vi "observacao_0MQ.vi"() -> ()   [LabVIEW 2012, in "Shared_160.lvlib"] (continued)
                  }
                }
                n2306 = case shown="True" w2937 {
                  tunnel: w2938 -> [_ w2940]
                  frame False {
                  }
                  frame True {
                    w2943 = u16 4 items=["ZERO", "AH", "DEC", "TUBO", "CUP"] ("Controlador")
                    n2307 = global write "Global_Telescopio.vi" "RevCupTO"(w2940) -> ()
                    n2308 = local write "StatDome"("Waiting" ("Status")) -> ()
                    n2309 = call "Monta Comando.vi"("Comando"="PARAR", "Dispositivo"="PROG", "Controlador"=w2943) -> ()  [unwired: 4 in, 3 out]
                  }
                }
              }
              frame Disabled {
                # "20240820"
                n2310 = global read "Global_Telescopio.vi" "RevCupTO"() -> (w2946:u32)
                n2311 = global read "Global_Telescopio.vi" "QtdEtiquetas"() -> (w2953:i16)
                n2312 = local read "DestCUP"() -> (w2952:i16)
                n2313 = Divide(x=w2953, y=2) -> (x/y=w2951:dbl)
                n2314 = call "TickTimeout.vi"("msInicial"=w2946, "msTimeout"=u32 3000) -> ("msTick"=w2949:u32, "Timeout"=w2948:bool)  [unwired: 1 out]
                n2315 = Subtract(x=w2952, y=w2951) -> (x-y=w2954:dbl)
                n2316 = Add(x=w2952, y=w2951) -> (x+y=w2955:dbl)
                n2317 = Greater?(x=w2955, y=w2953) -> (0:w2956:bool)
                n2318 = Select(t=w2954, s=w2956, f=w2955) -> (s? t:f=w2957:dbl)
                n2319 = case shown="True" w2948 {
                  tunnel: w2949 -> [_ w2964]
                  tunnel: w2957 -> [_ w2959]
                  frame False {
                  }
                  frame True {
                    w2963 = u16 4 items=["ZERO", "AH", "DEC", "TUBO", "CUP"] ("Controlador")
                    n2320 = To Word Integer(number=w2959) -> (16bit integer=w2958:i16)
                    n2321 = global write "Global_Telescopio.vi" "RevCupTO"(w2964) -> ()
                    n2322 = Number To Decimal String(number=w2958) -> (decimal integer string=w2961:string)  [unwired: 1 in]
                    n2323 = local write "StatDome"("Reverting" ("Status")) -> ()
                    n2324 = call "Monta Comando.vi"("Set Point"=w2961, "Comando"="MOVER" ("Dispositivo"), "Dispositivo"="DOMO", "Controlador"=w2963) -> ()  [unwired: 3 in, 3 out]
                  }
                }
              }
              frame Disabled {
                # "20240820"
                n2325 = global read "Global_Telescopio.vi" "RevCupTO"() -> (w2966:u32)
                n2326 = call "TickTimeout.vi"("msInicial"=w2966, "msTimeout"=u32 10000) -> ("msTick"=w2969:u32, "Timeout"=w2968:bool)  [unwired: 1 out]
                n2327 = case shown="True" w2968 {
                  tunnel: w2969 -> [_ w2970]
                  frame False {
                  }
                  frame True {
                    w2973 = u16 4 items=["ZERO", "AH", "DEC", "TUBO", "CUP"] ("Controlador")
                    n2328 = global write "Global_Telescopio.vi" "RevCupTO"(w2970) -> ()
                    n2329 = local write "StatDome"("Wait2s" ("Status")) -> ()
                    n2330 = call "Monta Comando.vi"("Comando"="PARAR", "Dispositivo"="PROG", "Controlador"=w2973) -> ()  [unwired: 4 in, 3 out]
                  }
                }
              }
              frame Disabled {
                n2331 = global read "Global_Telescopio.vi" "RevCupTO"() -> (w2975:u32)
                n2332 = call "TickTimeout.vi"("msInicial"=w2975, "msTimeout"=u32 2000) -> ("msTick"=w2978:u32, "Timeout"=w2977:bool)  [unwired: 1 out]
                n2333 = case shown="True" w2977 {
                  tunnel: w2978 -> [_ w2979]
                  frame False {
                  }
                  frame True {
                    n2334 = global write "Global_Telescopio.vi" "RevCupTO"(w2979) -> ()
                    n2335 = local write "StatDome"("Not Ready" ("Status")) -> ()
                  }
                }
              }
              frame Enabled {
              }
            }
            n2336 = global read "Global_Telescopio.vi" "Telescopio"() -> (w2917:bool)
            n2337 = local read "StatShutter"() -> (w2925:string)
            n2338 = local read "StatDome"() -> (w2927:string)
            n2339 = Select(t=1, s=w2917, f=2) -> (s? t:f=w2915:i32)
            n2340 = event shown="[2] \"BtDomeSTOP\": Value Change" {
              selector: _ -> [_ _ _ _ _ _ _ _]
              dyn-events: _ -> [_ _ _ _ _ _ _ _]
              timeout: 10 -> [_ _ _ _ _ _ _ _]
              tunnel: [FALSE ("NewVal") w3073 w3086 FALSE ("NewVal") FALSE ("NewVal") _ _ _] -> w2924
              tunnel: w2915 -> [_ w3072 _ _ _ _ _ _]
              event Timeout {
                n2341 = event-data() -> ()  [unwired: 1 in, 2 out]
              }
              event "BtDomeGO": Value Change {
                n2342 = event-data() -> ("NewVal"=w3074:bool)  [unwired: 1 in, 5 out]
                n2343 = local read "StatDome"() -> (w3077:string)
                n2344 = Equal?(x=w3077, y="Stopped" ("Status")) -> (x = y?=w3075:bool)
                n2345 = And(x=w3074, y=w3075) -> (x .and. y?=w3073:bool)
                n2346 = case shown="True" w3073 {
                  tunnel: w3072 -> [_ w3081]
                  frame False {
                  }
                  frame True {
                    # "20240820"
                    n2347 = local read "DomeNewPos"() -> (w3078:i32)
                    n2348 = Multiply(x=w3078, y=w3081) -> (x*y=w3079:i32)
                    n2349 = call "Checa destino cupula.vi"("Target"=w3079) -> ("moverCup"=w3080:bool)  [unwired: 6 in, 2 out]
                    n2350 = case shown="True" w3080 {
                      tunnel: w3079 -> [_ w3084]
                      frame False {
                      }
                      frame True {
                        # "Desabilita todas Abas"
                        n2351 = local write "DestCUP"(w3084) -> ()
                        n2352 = local write "DOME"(FALSE) -> ()
                        n2353 = property on="Setup, Pointing & Guiding" class="TabCtl (strict)"("Page Selector Visible"=FALSE) -> ()  [unwired: 2 in, 2 out]
                        n2354 = local write "StatDome"("Not Ready" ("Status")) -> ()
                      }
                    }
                  }
                }
              }
              event "BtDomeSTOP": Value Change {
                n2355 = event-data() -> ("NewVal"=w3086:bool)  [unwired: 1 in, 5 out]
                n2356 = case shown="True" w3086 {
                  frame False {
                  }
                  frame True {
                    n2357 = local read "StatDome"() -> (w3087:string)
                    n2358 = case shown="\"Moving\", Default" w3087 {
                      frame "Stopped" {
                      }
                      frame "Moving", Default {
                        w3088 = u16 4 items=["ZERO", "AH", "DEC", "TUBO", "CUP"] ("Controlador")
                        n2359 = local write "StatDome"("Stopping" ("Status")) -> ()
                        n2360 = call "Monta Comando.vi"("Comando"="PARAR", "Dispositivo"="PROG", "Controlador"=w3088) -> ()  [unwired: 4 in, 3 out]
                      }
                      frame "Not Ready" {
                        n2361 = local write "StatDome"("Stopped" ("Status")) -> ()
                      }
                    }
                  }
                }
              }
              event "BtShutOpen": Value Change {
                n2362 = event-data() -> ("NewVal"=w3095:bool)  [unwired: 1 in, 5 out]
                n2363 = local read "StatShutter"() -> (w3093:string)
                n2364 = case shown="True" w3095 {
                  tunnel: w3093 -> [_ w3096]
                  frame False {
                  }
                  frame True {
                    n2365 = case shown="\"Closed\"" w3096 {
                      frame "Opened", Default {
                      }
                      frame "Closed" {
                        w3097 = FALSE ("WeakSel")
                        w3098 = FALSE ("Coude")
                        w3099 = T5."Enabled" ("Disabled")
                        n2366 = property on="Coude" class="Bool (strict)"("DisabledEnum"=w3099) -> ()  [unwired: 2 in, 2 out]
                        n2367 = property on="Weak" class="Bool (strict)"("Disabled"=w3099) -> ()  [unwired: 2 in, 2 out]
                        n2368 = property on="Medium" class="Bool (strict)"("Disabled"=w3099) -> ()  [unwired: 2 in, 2 out]
                        n2369 = property on="Strong" class="Bool (strict)"("Disabled"=w3099) -> ()  [unwired: 2 in, 2 out]
                        n2370 = local write "StatShutter"("Busy to Open" ("Status")) -> ()
                        n2371 = local write "WeakSel"(w3097) -> ()
                        n2372 = local write "MediumSel"(w3097) -> ()
                        n2373 = local write "Coude"(w3098) -> ()
                        n2374 = local write "Weak"(w3098) -> ()
                        n2375 = local write "Medium"(w3098) -> ()
                        n2376 = local write "Strong"(w3098) -> ()
                        n2377 = local write "StrongSel"(w3097) -> ()
                        n2378 = local write "CoudeSel"(w3097) -> ()
                        n2379 = stacked-sequence {
                          frame #0 {
                            w3102 = u16 4 items=["ZERO", "AH", "DEC", "TUBO", "CUP"] ("Controlador")
                            n2380 = call "Monta Comando.vi"("Comando"="DESLIGAR", "Dispositivo"="FLAT_WEAK", "Controlador"=w3102) -> ()  [unwired: 4 in, 3 out]
                          }
                          frame #1 {
                            w3105 = u16 4 items=["ZERO", "AH", "DEC", "TUBO", "CUP"] ("Controlador")
                            n2381 = call "Monta Comando.vi"("Comando"="DESLIGAR", "Dispositivo"="FLAT_LO", "Controlador"=w3105) -> ()  [unwired: 4 in, 3 out]
                          }
                          frame #2 {
                            w3108 = u16 4 items=["ZERO", "AH", "DEC", "TUBO", "CUP"] ("Controlador")
                            n2382 = call "Monta Comando.vi"("Comando"="DESLIGAR", "Dispositivo"="FLAT_HI", "Controlador"=w3108) -> ()  [unwired: 4 in, 3 out]
                          }
                          frame #3 {
                            w3110 = u16 4 items=["ZERO", "AH", "DEC", "TUBO", "CUP"] ("Controlador")
                            n2383 = call "Monta Comando.vi"("Comando"="DESLIGAR", "Dispositivo"="FLAT_COUDE", "Controlador"=w3110) -> ()  [unwired: 4 in, 3 out]
                          }
                        }
                      }
                    }
                  }
                }
              }
              event "BtShutClose": Value Change {
                n2384 = event-data() -> ("NewVal"=w3114:bool)  [unwired: 1 in, 5 out]
                n2385 = case shown="True" w3114 {
                  frame False {
                  }
                  frame True {
                    n2386 = stacked-sequence {
                      frame #0 {
                        # "MUDANÇA:\nRemovido CASE que não setava essas\nvariáveis se StatShutter = Closed para\ngarantir fechamento da Trapeira."
                        n2387 = local write "DOME"(FALSE) -> ()
                        n2388 = local write "StatShutter"("Busy to Close" ("Status")) -> ()
                      }
                      frame #1 {
                        # "Escreve no LOG o estado do shutter"
                        # "Timer para escrever no log\ne enviar comando:\nCUP TRAPEIRA PARAR"
                        n2389 = Tick Count (ms)() -> (millisecond timer value=w3117:u32)
                        n2390 = local write "shutterTimeOld"(w3117) -> ()
                        n2391 = local write "timeStatShutterAlert"(w3117) -> ()
                        n2392 = local write "sendCommandShutter"(TRUE ("writeShutterLog")) -> ()
                        n2393 = call "Log_Shutter.vi"("command"=" ", "domeState"="CLOSED " ("command"), "pathLogDomeFile"="C:\\TCS\\LOG\\SHUTTER\\SHUTTER.TXT" ("pathLogFocoString")) -> ()  [unwired: 6 in]
                      }
                    }
                  }
                }
              }
              event "BtParavUp": Value Change {
                n2394 = event-data() -> ("NewVal"=w3122:bool)  [unwired: 1 in, 5 out]
                n2395 = case shown="True" w3122 {
                  frame False {
                  }
                  frame True {
                    w3125 = u16 4 items=["ZERO", "AH", "DEC", "TUBO", "CUP"] ("Controlador")
                    n2396 = call "Monta Comando.vi"("Comando"="SUBIR", "Dispositivo"="PARAVENTO" ("Comando"), "Controlador"=w3125) -> ()  [unwired: 4 in, 3 out]
                  }
                }
              }
              event "BtParavDown": Value Change {
                n2397 = event-data() -> ("NewVal"=w3126:bool)  [unwired: 1 in, 5 out]
                n2398 = case shown="True" w3126 {
                  frame False {
                  }
                  frame True {
                    w3129 = u16 4 items=["ZERO", "AH", "DEC", "TUBO", "CUP"] ("Controlador")
                    n2399 = call "Monta Comando.vi"("Comando"="DESCER", "Dispositivo"="PARAVENTO" ("Comando"), "Controlador"=w3129) -> ()  [unwired: 4 in, 3 out]
                  }
                }
              }
              event "BtParavStop": Value Change {
                n2400 = event-data() -> ("NewVal"=w3130:bool)  [unwired: 1 in, 5 out]
                n2401 = case shown="True" w3130 {
                  frame False {
                  }
                  frame True {
                    w3133 = u16 4 items=["ZERO", "AH", "DEC", "TUBO", "CUP"] ("Controlador")
                    n2402 = call "Monta Comando.vi"("Comando"="PARAR", "Dispositivo"="PARAVENTO" ("Comando"), "Controlador"=w3133) -> ()  [unwired: 4 in, 3 out]
                  }
                }
              }
            }
            n2403 = call "Bit Status CUP.vi"("NomeStatus"=w2926) -> ("StatBit"=w2923:bool)
            n2404 = global read "Global_Telescopio.vi" "PosCUP"() -> (w2919:i16)
            n2405 = case shown="\"Moving\"" w2927 {
              tunnel: w2923 -> [_ _ w3062 w3068]
              tunnel: w2924 -> [_ _ _ _]
              frame "", Default {
              }
              frame "Not Ready" {
                n2406 = local read "DestCUP"() -> (w3048:i16)
                n2407 = global read "Global_Telescopio.vi" "PosCUP"() -> (w3050:i16)
                n2408 = call "TickTimeout.vi"() -> ("msTick"=w3051:u32)  [unwired: 2 in, 2 out]
                n2409 = call "Checa destino cupula.vi"("Target"=w3048) -> ("moverCup"=w3047:bool, "angTarget"=w3049:string)  [unwired: 6 in, 1 out]
                n2410 = case shown="True" w3047 {
                  tunnel: w3051 -> [_ w3057]
                  tunnel: w3050 -> [_ w3056]
                  tunnel: w3049 -> [_ w3055]
                  tunnel: w3048 -> [_ w3054]
                  frame False {
                    n2411 = local write "StatDome"("Stopping" ("Status")) -> ()
                  }
                  frame True {
                    w3061 = u16 4 items=["ZERO", "AH", "DEC", "TUBO", "CUP"] ("Controlador")
                    # "20240820"
                    n2412 = global write "Global_Telescopio.vi" "RevCupTO"(w3057) -> ()
                    n2413 = local write "TargetCup"(w3055) -> ()
                    n2414 = global write "Global_Telescopio.vi" "CupStartPos"(w3056) -> ()
                    n2415 = Number To Decimal String(number=w3054) -> (decimal integer string=w3058:string)  [unwired: 1 in]
                    n2416 = local write "StatDome"("Moving" ("Status")) -> ()
                    n2417 = call "Monta Comando.vi"("Set Point"=w3058, "Comando"="MOVER", "Dispositivo"="DOMO" ("Comando"), "Controlador"=w3061) -> ()  [unwired: 3 in, 3 out]
                  }
                }
              }
              frame "Moving" {
                n2418 = case shown="False" w3062 {
                  frame False {
                    n2419 = local read "DestCUP"() -> (w3067:i16)
                    n2420 = call "Checa destino cupula.vi"("Target"=w3067) -> ("moverCup"=w3066:bool)  [unwired: 6 in, 2 out]
                    n2421 = Select(t="Not Ready" ("Comando"), s=w3066, f="Stopping" ("Comando")) -> (s? t:f=w3065:string)
                    n2422 = local write "StatDome"(w3065) -> ()
                  }
                  frame True {
                  }
                }
              }
              frame "Stopping" {
                n2423 = case shown="False" w3068 {
                  frame False {
                    # "Reabilita Abas"
                    n2424 = property on="Setup, Pointing & Guiding" class="TabCtl (strict)"("Page Selector Visible"=TRUE) -> ()  [unwired: 2 in, 2 out]
                    n2425 = local write "StatDome"("Stopped" ("Status")) -> ()
                  }
                  frame True {
                  }
                }
              }
            }
            n2426 = call "Bit Status CUP.vi"("NomeStatus"=w2922) -> ("StatBit"=w2921:bool)
            "LedShutter" <- w2921
            n2427 = case shown="\"Busy to Close\"" w2925 {
              tunnel: w2924 -> [_ _ _ _]
              tunnel: w2923 -> [_ w3030 w3036 _]
              frame "", Default {
              }
              frame "Busy to Open" {
                n2428 = case shown="False" w3030 {
                  frame False {
                    w3034 = u16 4 items=["ZERO", "AH", "DEC", "TUBO", "CUP"] ("Controlador")
                    n2429 = call "TickTimeout.vi"() -> ("msTick"=w3031:u32)  [unwired: 2 in, 2 out]
                    n2430 = local write "TimeoutTrap"(w3031) -> ()
                    n2431 = local write "StatShutter"("Moving" ("Status")) -> ()
                    n2432 = call "Monta Comando.vi"("Comando"="ABRIR", "Dispositivo"="TRAPEIRA" ("Comando"), "Controlador"=w3034) -> ()  [unwired: 4 in, 3 out]
                  }
                  frame True {
                  }
                }
              }
              frame "Busy to Close" {
                n2433 = case shown="False" w3036 {
                  frame False {
                    w3040 = u16 4 items=["ZERO", "AH", "DEC", "TUBO", "CUP"] ("Controlador")
                    n2434 = call "TickTimeout.vi"() -> ("msTick"=w3037:u32)  [unwired: 2 in, 2 out]
                    n2435 = local write "TimeoutTrap"(w3037) -> ()
                    n2436 = local write "StatShutter"("Moving" ("Status")) -> ()
                    n2437 = call "Monta Comando.vi"("Comando"="FECHAR", "Dispositivo"="TRAPEIRA" ("Comando"), "Controlador"=w3040) -> ()  [unwired: 4 in, 3 out]
                  }
                  frame True {
                  }
                }
              }
              frame "Moving" {
                n2438 = local read "TimeoutTrap"() -> (w3042:u32)
                n2439 = call "TickTimeout.vi"("msInicial"=w3042, "msTimeout"=u32 12000) -> ("Timeout"=w3043:bool)  [unwired: 2 out]
                n2440 = case shown="False" w3043 {
                  selector: w3043 -> [w3046 _]
                  frame False {
                    n2441 = Not(x=w3046) -> (.not. x?=w3045:bool)
                    n2442 = local write "RefreshShutterState"(w3045) -> ()
                  }
                  frame True {
                  }
                }
              }
            }
            n2443 = local read "RefreshShutterState"() -> (w2920:bool)
            n2444 = Divide(x=w2919, y=w2915) -> (x/y=w2930:dbl)
            n2445 = To Word Integer(number=w2930) -> (16bit integer=→"AngCup":i16)
            n2446 = case shown="True" w2920 {
              selector: w2920 -> [_ w3025]
              tunnel: w2921 -> [_ w3026]
              frame False {
              }
              frame True {
                n2447 = Not(x=w3025) -> (.not. x?=→"RefreshShutterState":bool)
                n2448 = Select(t="Opened" ("Status"), s=w3026, f="Closed" ("Status")) -> (s? t:f=w3027:string)
                n2449 = local write "StatShutter"(w3027) -> ()
              }
            }
            n2450 = local read "Flag-ShutClose"() -> (w2913:bool)
            n2451 = local read "Flag-ShutOpen"() -> (w2912:bool)
            n2452 = event shown="[1] \"BtShutClose\": Value Change" {
              selector: _ -> [_ _ _]
              dyn-events: _ -> [_ _ _]
              timeout: 10 -> [_ _ _]
              event Timeout {
                n2453 = event-data() -> ()  [unwired: 1 in, 2 out]
              }
              event "BtShutClose": Value Change {
                # "Desabilita todas Abas"
                n2454 = event-data() -> ("NewVal"=w3006:bool)  [unwired: 1 in, 4 out]
                n2455 = case shown="True" w3006 {
                  selector: w3006 -> [_ w3011]
                  frame False {
                  }
                  frame True {
                    n2456 = Get Date/Time In Seconds() -> (seconds since 1Jan1904=w3010:timestamp)
                    n2457 = Add(x=w3010, y=10.0) -> (x+y=w3008:timestamp)
                    n2458 = local write "Cont-ShutOpen"(w3008) -> ()
                    n2459 = property on="Setup, Pointing & Guiding" class="TabCtl (strict)"("Page Selector Visible"=FALSE) -> ()  [unwired: 2 in, 2 out]
                    "Flag-ShutClose" <- w3011
                  }
                }
              }
              event "BtShutOpen": Value Change {
                # "Desabilita todas Abas"
                n2460 = event-data() -> ("NewVal"=w3012:bool)  [unwired: 1 in, 4 out]
                n2461 = case shown="True" w3012 {
                  selector: w3012 -> [_ w3013]
                  frame False {
                  }
                  frame True {
                    n2462 = stacked-sequence {
                      tunnel: w3013 -> [w3018 _]
                      frame #0 {
                        n2463 = Get Date/Time In Seconds() -> (seconds since 1Jan1904=w3017:timestamp)
                        n2464 = Add(x=w3017, y=10.0) -> (x+y=→"Cont-ShutOpen":timestamp)
                        n2465 = property on="Setup, Pointing & Guiding" class="TabCtl (strict)"("Page Selector Visible"=FALSE) -> ()  [unwired: 2 in, 2 out]
                        "Flag-ShutOpen" <- w3018
                      }
                      frame #1 {
                        # "Escreve no LOG o estado do shutter"
                        # "Timer para escrever no log\ne enviar comando:\nCUP TRAPEIRA PARAR"
                        n2466 = Tick Count (ms)() -> (millisecond timer value=w3019:u32)
                        n2467 = local write "sendCommandShutter"(TRUE ("writeShutterLog")) -> ()
                        n2468 = local write "timeStatShutterAlert"(w3019) -> ()
                        n2469 = local write "shutterTimeOld"(w3019) -> ()
                        n2470 = call "Log_Shutter.vi"("command"=" ", "domeState"="OPENED " ("command"), "pathLogDomeFile"="C:\\TCS\\LOG\\SHUTTER\\SHUTTER.TXT" ("pathLogFocoString")) -> ()  [unwired: 6 in]
                      }
                    }
                  }
                }
              }
            }
            n2471 = event shown="[4] \"CW\": Mouse Up" {
              selector: _ -> [_ _ _ _ _]
              dyn-events: _ -> [_ _ _ _ _]
              timeout: 100 -> [_ _ _ _ _]
              event Timeout {
                n2472 = event-data() -> ()  [unwired: 1 in, 2 out]
              }
              event "CCW": Mouse Down {
                w2981 = "GIRAR_CCW" ("Comando")
                w2982 = u16 4 items=["ZERO", "AH", "DEC", "TUBO", "CUP"] ("Controlador")
                # "Envia o comando GIRAR"
                n2473 = event-data() -> ()  [unwired: 1 in, 7 out]
                n2474 = local write "Command"(w2981) -> ()
                n2475 = call "Monta Comando.vi"("Comando"=w2981, "Dispositivo"="DOMO" ("Comando"), "Controlador"=w2982) -> ()  [unwired: 4 in, 3 out]
              }
              event "CCW": Mouse Up {
                n2476 = event-data() -> ()  [unwired: 1 in, 7 out]
                n2477 = stacked-sequence {
                  frame #0 {
                    w2984 = "PARAR" ("Comando")
                    w2985 = u16 4 items=["ZERO", "AH", "DEC", "TUBO", "CUP"] ("Controlador")
                    # "Envia o comando PARAR"
                    n2478 = local write "Command"(w2984) -> ()
                    n2479 = call "Monta Comando.vi"("Comando"=w2984, "Dispositivo"="DOMO" ("Comando"), "Controlador"=w2985) -> ()  [unwired: 4 in, 3 out]
                  }
                  frame #1 {
                    n2480 = Wait (ms)(milliseconds to wait=u32 100) -> ()  [unwired: 1 out]
                  }
                  frame #2 {
                    w2988 = "PARAR" ("Comando")
                    w2989 = u16 4 items=["ZERO", "AH", "DEC", "TUBO", "CUP"] ("Controlador")
                    # "Envia o comando PARAR"
                    n2481 = local write "Command"(w2988) -> ()
                    n2482 = call "Monta Comando.vi"("Comando"=w2988, "Dispositivo"="DOMO" ("Comando"), "Controlador"=w2989) -> ()  [unwired: 4 in, 3 out]
                  }
                }
              }
              event "CW": Mouse Down {
                w2991 = "GIRAR_CW" ("Comando")
                w2992 = u16 4 items=["ZERO", "AH", "DEC", "TUBO", "CUP"] ("Controlador")
                # "Envia o comando GIRAR"
                n2483 = event-data() -> ()  [unwired: 1 in, 7 out]
                n2484 = local write "Command"(w2991) -> ()
                n2485 = call "Monta Comando.vi"("Comando"=w2991, "Dispositivo"="DOMO" ("Comando"), "Controlador"=w2992) -> ()  [unwired: 4 in, 3 out]
              }
              event "CW": Mouse Up {
                n2486 = event-data() -> ()  [unwired: 1 in, 7 out]
                n2487 = stacked-sequence {
                  frame #0 {
                    w2994 = "PARAR" ("Comando")
                    w2995 = u16 4 items=["ZERO", "AH", "DEC", "TUBO", "CUP"] ("Controlador")
                    # "Envia o comando PARAR"
                    n2488 = local write "Command"(w2994) -> ()
                    n2489 = call "Monta Comando.vi"("Comando"=w2994, "Dispositivo"="DOMO" ("Comando"), "Controlador"=w2995) -> ()  [unwired: 4 in, 3 out]
                  }
                  frame #1 {
                    n2490 = Wait (ms)(milliseconds to wait=u32 100) -> ()  [unwired: 1 out]
                  }
                  frame #2 {
                    w2998 = "PARAR" ("Comando")
                    w2999 = u16 4 items=["ZERO", "AH", "DEC", "TUBO", "CUP"] ("Controlador")
                    # "Envia o comando PARAR"
                    n2491 = local write "Command"(w2998) -> ()
                    n2492 = call "Monta Comando.vi"("Comando"=w2998, "Dispositivo"="DOMO" ("Comando"), "Controlador"=w2999) -> ()  [unwired: 4 in, 3 out]
                  }
                }
              }
            }
            n2493 = Or(x=w2913, y=w2912) -> (x .or. y?=w2911:bool)
            n2494 = case shown="True" w2911 {
              frame False {
              }
              frame True {
                n2495 = local read "Cont-ShutOpen"() -> (w3002:timestamp)
                n2496 = Get Date/Time In Seconds() -> (seconds since 1Jan1904=w3003:timestamp)
                n2497 = Greater Or Equal?(x=w3003, y=w3002) -> (x >= y?=w3001:bool)
                n2498 = case shown="True" w3001 {
                  frame False {
                  }
                  frame True {
                    w3005 = FALSE ("Flag-ShutClose")
                    # "Reabilita todas Abas"
                    n2499 = local write "Flag-ShutClose"(w3005) -> ()
                    n2500 = local write "Flag-ShutOpen"(w3005) -> ()
                    n2501 = property on="Setup, Pointing & Guiding" class="TabCtl (strict)"("Page Selector Visible"=TRUE) -> ()  [unwired: 2 in, 2 out]
                  }
                }
              }
            }
            "Command" <- "" ("Command")
          }
          frame "UTILS " {
            n2502 = stacked-sequence {
              frame #0 {
                # "Acionamento das Abas do\nEspelho\n\nComandos sempre precedidos\nde ESPAÇO\n\nTUBO TAMPAS ESCREVER = 80 80\n\nLigar power geral       08 08\nDesligar power geral  08 00\nLigar System              10 10\nDesligar System         10 00\nPassar para Remoto  20 20\nPassar para Local      20 00\nSel. device central     40 40\nSel. device bowl         40 00\nAction open                80 80\nAction close                80 00"
                n2503 = event shown="[1] \"MODE\": Value Change" {
                  selector: _ -> [_ _ _]
                  dyn-events: _ -> [_ _ _]
                  timeout: 10 -> [_ _ _]
                  event Timeout {
                    n2504 = event-data() -> ()  [unwired: 1 in, 2 out]
                  }
                  event "MODE": Value Change {
                    n2505 = event-data() -> ("NewVal"=w3148:bool)  [unwired: 1 in, 5 out]
                    "LED MODE" <- w3148
                    n2506 = case shown="False" w3148 {
                      frame False {
                        w3153 = u16 3 items=["ZERO", "AH", "DEC", "TUBO", "CUP"] ("Controlador")
                        # "DESABILITA"
                        # "APENAS PASSANDO COMANDO PARA MANETE"
                        # "MODE E GERAL = 0"
                        # "MODE HADSET"
                        n2507 = call "Monta Comando.vi"("Set Point"=" F8 90", "Comando"="ESCREVER", "Dispositivo"="TAMPAS" ("Comando"), "Controlador"=w3153) -> ()  [unwired: 3 in, 3 out]
                        n2508 = property on="ACTION" class="Bool (strict)"("Disabled"=u8 2) -> ()  [unwired: 2 in, 2 out]
                      }
                      frame True {
                        w3158 = u16 3 items=["ZERO", "AH", "DEC", "TUBO", "CUP"] ("Controlador")
                        # "HABILITA"
                        # "APENAS PASSANDO COMOANDO PARA TCSPD"
                        # "MODE E GERAL = 1"
                        # "MODE TCSPD"
                        n2509 = call "Monta Comando.vi"("Set Point"=" 48 48", "Comando"="ESCREVER", "Dispositivo"="TAMPAS" ("Comando"), "Controlador"=w3158) -> ()  [unwired: 3 in, 3 out]
                        n2510 = property on="ACTION" class="Bool (strict)"("Disabled"=u8 0) -> ()  [unwired: 2 in, 2 out]
                      }
                    }
                  }
                  event "ACTION": Value Change {
                    n2511 = event-data() -> ("NewVal"=w3159:bool)  [unwired: 1 in, 5 out]
                    n2512 = case shown="False" w3159 {
                      frame False {
                        # "FECHAR"
                        n2513 = local write "ESTADO FECHAR"("INICIO" ("ESTADO ABRIR")) -> ()
                        n2514 = local write "ESTADO ABRIR"("REPOUSO" ("ESTADO ABRIR")) -> ()
                      }
                      frame True {
                        # "ABRIR"
                        n2515 = local write "ESTADO FECHAR"("REPOUSO" ("ESTADO ABRIR")) -> ()
                        n2516 = local write "ESTADO ABRIR"("INICIO" ("ESTADO ABRIR")) -> ()
                      }
                    }
                  }
                }
                n2517 = Tick Count (ms)() -> (millisecond timer value=w3139:u32)
                n2518 = Greater Or Equal?(x=w3139, y="TIMER TICK") -> (x >= y?=w3135:bool)
                n2519 = And(x=w3135, y=FALSE) -> (x .and. y?=w3136:bool)
                n2520 = case shown="True" w3136 {
                  frame False {
                  }
                  frame True {
                    w3172 = u16 3 items=["ZERO", "AH", "DEC", "TUBO", "CUP", "CASS", "COUDE"] ("Controlador")
                    # "2 SEGUNDOS"
                    n2521 = Tick Count (ms)() -> (millisecond timer value=w3169:u32)
                    n2522 = Add(x=w3169, y=u32 10000) -> (x+y=w3167:u32)
                    n2523 = call "Status_das_Tampas.vi"("Controlador"=w3172, "DISPOSITIVO"="TAMPAS", "Comando"="LER") -> ("Fechado/Aberto"=w3166:bool, "Dispositivo Bacia/Centar"=w3165:bool)  [unwired: 6 in, 5 out]
                    n2524 = local write "TIMER TICK"(w3167) -> ()
                    n2525 = Not(x=w3166) -> (.not. x?=w3164:bool)
                    n2526 = And(x=w3164, y=w3165) -> ()  [unwired: 1 out]
                  }
                }
                n2527 = event shown="[4] \"FLAT-FIELD\": Value Change" {
                  selector: _ -> [_ _ _ _ _ _]
                  dyn-events: _ -> [_ _ _ _ _ _]
                  timeout: 10 -> [_ _ _ _ _ _]
                  event Timeout {
                    n2528 = event-data() -> ()  [unwired: 1 in, 2 out]
                  }
                  event "BtUtilPark": Value Change {
                    n2529 = event-data() -> ("NewVal"=w3173:bool)  [unwired: 1 in, 5 out]
                    n2530 = case shown="True" w3173 {
                      frame False {
                      }
                      frame True {
                        w3176 = u16 4 items=["ZERO", "AH", "DEC", "TUBO", "CUP"] ("Controlador")
                        w3177 = FALSE ("MOUNT")
                        w3180 = 0 ("M_AH")
                        w3181 = u8 2 ("Disabled")
                        w3178 = FALSE ("Page Selector Visible")
                        w3185 = 1 ("M_AH")
                        # "Carrega Parâmetros da Configuração"
                        # "Seta Máq GO"
                        # "Desabilita todas Abas"
                        # "DESABILITA TODOS"
                        n2531 = local write "DOME"(w3178) -> ()
                        n2532 = property on="Setup, Pointing & Guiding" class="TabCtl (strict)"("Page Selector Visible"=w3178) -> ()  [unwired: 2 in, 2 out]
                        n2533 = local write "statAH"(w3180) -> ()
                        n2534 = local write "statCUP"(w3180) -> ()
                        n2535 = local write "statDEC"(w3180) -> ()
                        n2536 = local write "M_DEC"(w3185) -> ()
                        n2537 = local write "M_AH"(w3185) -> ()
                        n2538 = local write "M_CUP"(w3185) -> ()
                        n2539 = global read "Global_Telescopio.vi" "DestDEC"() -> (w3183:dbl)
                        n2540 = global read "Global_Telescopio.vi" "DestCUP"() -> (w3182:i32)
                        n2541 = global read "Global_Telescopio.vi" "DestAH"() -> (w3184:dbl)
                        n2542 = property on="BtUtilPark" class="Bool (strict)"("Disabled"=w3181) -> ()  [unwired: 2 in, 2 out]
                        n2543 = property on="ECASS" class="Bool (strict)"("Disabled"=w3181) -> ()  [unwired: 2 in, 2 out]
                        n2544 = local write "DestAH"(w3184) -> ()
                        n2545 = local write "DestCUP"(w3182) -> ()
                        n2546 = local write "DestDEC"(w3183) -> ()
                        n2547 = global write "Global_Telescopio.vi" "Parking"(TRUE ("Page Selector Visible")) -> ()
                        n2548 = property on="BtUtilZenith" class="Bool (strict)"("Disabled"=w3181) -> ()  [unwired: 2 in, 2 out]
                        n2549 = property on="FLAT-FIELD" class="Bool (strict)"("Disabled"=w3181) -> ()  [unwired: 2 in, 2 out]
                        n2550 = property on="PROTEÇÃO" class="Bool (strict)"("Disabled"=w3181) -> ()  [unwired: 2 in, 2 out]
                        n2551 = local write "MOUNT"(w3177) -> ()
                        n2552 = local write "GUIDER"(w3177) -> ()
                        n2553 = call "Monta Comando.vi"("Comando"="LIGAR", "Dispositivo"="LAMP_CAM" ("Comando"), "Controlador"=w3176) -> ()  [unwired: 4 in, 3 out]
                      }
                    }
                  }
                  event "BtUtilZenith": Value Change {
                    n2554 = event-data() -> ("NewVal"=w3186:bool)  [unwired: 1 in, 5 out]
                    n2555 = case shown="True" w3186 {
                      frame False {
                      }
                      frame True {
                        w3189 = u16 4 items=["ZERO", "AH", "DEC", "TUBO", "CUP"] ("Controlador")
                        w3190 = FALSE ("MOUNT")
                        w3193 = 0 ("M_AH")
                        w3194 = u8 2 ("Disabled")
                        w3192 = FALSE ("Page Selector Visible")
                        w3198 = 1 ("M_AH")
                        # "Seta Máq GO"
                        # "Desabilita todas Abas"
                        # "DESABILITA TODOS"
                        n2556 = local write "M_DEC"(w3198) -> ()
                        n2557 = local write "M_AH"(w3198) -> ()
                        n2558 = local write "M_CUP"(w3198) -> ()
                        n2559 = local write "DOME"(w3192) -> ()
                        n2560 = property on="Setup, Pointing & Guiding" class="TabCtl (strict)"("Page Selector Visible"=w3192) -> ()  [unwired: 2 in, 2 out]
                        n2561 = call "Monta Comando.vi"("Comando"="LIGAR", "Dispositivo"="LAMP_CAM" ("Comando"), "Controlador"=w3189) -> ()  [unwired: 4 in, 3 out]
                        n2562 = local write "statAH"(w3193) -> ()
                        n2563 = local write "statCUP"(w3193) -> ()
                        n2564 = local write "statDEC"(w3193) -> ()
                        n2565 = global read "Global_Telescopio.vi" "Telescopio"() -> (w3191:bool)
                        n2566 = property on="BtUtilPark" class="Bool (strict)"("Disabled"=w3194) -> ()  [unwired: 2 in, 2 out]
                        n2567 = property on="ECASS" class="Bool (strict)"("Disabled"=w3194) -> ()  [unwired: 2 in, 2 out]
                        n2568 = case shown="False" w3191 {
                          tunnel: [0.0 ("DestAH") 0.0 ("DestAH")] -> w3197
                          tunnel: [-0.3933 ("DestDEC") -0.3933 ("DestDEC")] -> w3196
                          tunnel: [i16 98 ("DestCUP") i16 80 ("DestCUP")] -> w3195
                          frame False {
                          }
                          frame True {
                          }
                        }
                        n2569 = property on="BtUtilZenith" class="Bool (strict)"("Disabled"=w3194) -> ()  [unwired: 2 in, 2 out]
                        n2570 = property on="FLAT-FIELD" class="Bool (strict)"("Disabled"=w3194) -> ()  [unwired: 2 in, 2 out]
                        n2571 = local write "DestAH"(w3197) -> ()
                        n2572 = local write "DestCUP"(w3195) -> ()
                        n2573 = local write "DestDEC"(w3196) -> ()
                        n2574 = property on="PROTEÇÃO" class="Bool (strict)"("Disabled"=w3194) -> ()  [unwired: 2 in, 2 out]
                        n2575 = local write "MOUNT"(w3190) -> ()
                        n2576 = local write "GUIDER"(w3190) -> ()
                      }
                    }
                  }
                  event "ECASS": Value Change {
                    n2577 = event-data() -> ("NewVal"=w3205:bool)  [unwired: 1 in, 5 out]
                    n2578 = case shown="True" w3205 {
                      frame False {
                      }
                      frame True {
                        w3208 = u16 4 items=["ZERO", "AH", "DEC", "TUBO", "CUP"] ("Controlador")
                        w3209 = FALSE ("MOUNT")
                        w3212 = 0 ("M_AH")
                        w3213 = u8 2 ("Disabled")
                        w3211 = FALSE ("Page Selector Visible")
                        w3217 = 1 ("M_AH")
                        # "Seta Máq GO"
                        # "Desabilita todas Abas"
                        # "DESABILITA TODOS"
                        n2579 = local write "M_DEC"(w3217) -> ()
                        n2580 = local write "M_AH"(w3217) -> ()
                        n2581 = local write "M_CUP"(w3217) -> ()
                        n2582 = local write "DOME"(w3211) -> ()
                        n2583 = property on="Setup, Pointing & Guiding" class="TabCtl (strict)"("Page Selector Visible"=w3211) -> ()  [unwired: 2 in, 2 out]
                        n2584 = local write "statAH"(w3212) -> ()
                        n2585 = local write "statCUP"(w3212) -> ()
                        n2586 = local write "statDEC"(w3212) -> ()
                        n2587 = call "Monta Comando.vi"("Comando"="LIGAR", "Dispositivo"="LAMP_CAM" ("Comando"), "Controlador"=w3208) -> ()  [unwired: 4 in, 3 out]
                        n2588 = global read "Global_Telescopio.vi" "Telescopio"() -> (w3210:bool)
                        n2589 = property on="BtUtilPark" class="Bool (strict)"("Disabled"=w3213) -> ()  [unwired: 2 in, 2 out]
                        n2590 = property on="ECASS" class="Bool (strict)"("Disabled"=w3213) -> ()  [unwired: 2 in, 2 out]
                        n2591 = property on="BtUtilZenith" class="Bool (strict)"("Disabled"=w3213) -> ()  [unwired: 2 in, 2 out]
                        n2592 = property on="FLAT-FIELD" class="Bool (strict)"("Disabled"=w3213) -> ()  [unwired: 2 in, 2 out]
                        n2593 = case shown="False" w3210 {
                          tunnel: [0.0 ("DestAH") 0.0 ("DestAH")] -> w3216
                          tunnel: [0.4 ("DestDEC") 0.4 ("DestDEC")] -> w3215
                          tunnel: [i16 98 ("DestCUP") i16 80 ("DestCUP")] -> w3214
                          frame False {
                          }
                          frame True {
                          }
                        }
                        n2594 = property on="PROTEÇÃO" class="Bool (strict)"("Disabled"=w3213) -> ()  [unwired: 2 in, 2 out]
                        n2595 = local write "GUIDER"(w3209) -> ()
                        n2596 = local write "MOUNT"(w3209) -> ()
                        n2597 = local write "DestAH"(w3216) -> ()
                        n2598 = local write "DestCUP"(w3214) -> ()
                        n2599 = local write "DestDEC"(w3215) -> ()
                      }
                    }
                  }
                  event "FLAT-FIELD": Value Change {
                    n2600 = event-data() -> ("NewVal"=w3224:bool)  [unwired: 1 in, 5 out]
                    n2601 = case shown="True" w3224 {
                      frame False {
                      }
                      frame True {
                        w3227 = u16 4 items=["ZERO", "AH", "DEC", "TUBO", "CUP"] ("Controlador")
                        w3228 = FALSE ("MOUNT")
                        w3230 = 0 ("M_AH")
                        w3232 = u8 2 ("Disabled")
                        w3231 = FALSE ("Page Selector Visible")
                        w3236 = 1 ("M_AH")
                        # "Seta Máq GO"
                        # "Desabilita todas Abas"
                        # "DESABILITA TODOS"
                        n2602 = local write "M_DEC"(w3236) -> ()
                        n2603 = local write "M_AH"(w3236) -> ()
                        n2604 = local write "M_CUP"(w3236) -> ()
                        n2605 = local write "DOME"(w3231) -> ()
                        n2606 = property on="Setup, Pointing & Guiding" class="TabCtl (strict)"("Page Selector Visible"=w3231) -> ()  [unwired: 2 in, 2 out]
                        n2607 = call "Monta Comando.vi"("Comando"="LIGAR", "Dispositivo"="LAMP_CAM" ("Comando"), "Controlador"=w3227) -> ()  [unwired: 4 in, 3 out]
                        n2608 = local write "statAH"(w3230) -> ()
                        n2609 = local write "statCUP"(w3230) -> ()
                        n2610 = local write "statDEC"(w3230) -> ()
                        n2611 = global read "Global_Telescopio.vi" "Telescopio"() -> (w3229:bool)
                        n2612 = property on="BtUtilPark" class="Bool (strict)"("Disabled"=w3232) -> ()  [unwired: 2 in, 2 out]
                        n2613 = property on="ECASS" class="Bool (strict)"("Disabled"=w3232) -> ()  [unwired: 2 in, 2 out]
                        n2614 = case shown="False" w3229 {
                          tunnel: [0.0715 ("DestAH") 0.31416 ("DestAH")] -> w3235
                          tunnel: [0.641 ("DestDEC") -0.39415 ("DestDEC")] -> w3234
                          tunnel: [i16 306 ("DestCUP") i16 133 ("DestCUP")] -> w3233
                          frame False {
                          }
                          frame True {
                          }
                        }
                        n2615 = property on="BtUtilZenith" class="Bool (strict)"("Disabled"=w3232) -> ()  [unwired: 2 in, 2 out]
                        n2616 = property on="FLAT-FIELD" class="Bool (strict)"("Disabled"=w3232) -> ()  [unwired: 2 in, 2 out]
                        n2617 = local write "DestAH"(w3235) -> ()
                        n2618 = local write "DestCUP"(w3233) -> ()
                        n2619 = local write "DestDEC"(w3234) -> ()
                        n2620 = property on="PROTEÇÃO" class="Bool (strict)"("Disabled"=w3232) -> ()  [unwired: 2 in, 2 out]
                        n2621 = local write "GUIDER"(w3228) -> ()
                        n2622 = local write "MOUNT"(w3228) -> ()
                      }
                    }
                  }
                  event "PROTEÇÃO": Value Change {
                    n2623 = event-data() -> ("NewVal"=w3243:bool)  [unwired: 1 in, 5 out]
                    n2624 = case shown="True" w3243 {
                      frame False {
                      }
                      frame True {
                        w3244 = FALSE ("MOUNT")
                        w3246 = 0 ("M_AH")
                        w3245 = FALSE ("Page Selector Visible")
                        w3248 = u8 2 ("Disabled")
                        # "Seta Máq GO"
                        # "Desabilita todas Abas"
                        # "DESABILITA TODOS"
                        n2625 = local write "DOME"(w3245) -> ()
                        n2626 = property on="Setup, Pointing & Guiding" class="TabCtl (strict)"("Page Selector Visible"=w3245) -> ()  [unwired: 2 in, 2 out]
                        n2627 = local write "statAH"(w3246) -> ()
                        n2628 = local write "statCUP"(w3246) -> ()
                        n2629 = local write "statDEC"(w3246) -> ()
                        n2630 = property on="BtUtilPark" class="Bool (strict)"("Disabled"=w3248) -> ()  [unwired: 2 in, 2 out]
                        n2631 = property on="ECASS" class="Bool (strict)"("Disabled"=w3248) -> ()  [unwired: 2 in, 2 out]
                        n2632 = property on="BtUtilZenith" class="Bool (strict)"("Disabled"=w3248) -> ()  [unwired: 2 in, 2 out]
                        n2633 = property on="FLAT-FIELD" class="Bool (strict)"("Disabled"=w3248) -> ()  [unwired: 2 in, 2 out]
                        n2634 = local write "M_PROT"(1 ("M_PROT")) -> ()
                        n2635 = local write "GUIDER"(w3244) -> ()
                        n2636 = local write "MOUNT"(w3244) -> ()
                        n2637 = property on="PROTEÇÃO" class="Bool (strict)"("Disabled"=w3248) -> ()  [unwired: 2 in, 2 out]
                      }
                    }
                  }
                }
                n2638 = case shown="True" "STOP" {
                  frame False {
                  }
                  frame True {
                    n2639 = stacked-sequence {
                      frame #0 {
                        w3250 = 0 ("estado")
                        # "Zera Máquina de Estado\nPelo Botão STOP"
                        n2640 = property on="Setup, Pointing & Guiding" class="TabCtl (strict)"("Page Selector Visible"=TRUE) -> ()  [unwired: 2 in, 2 out]
                        n2641 = call "Stop.vi"() -> ()  [unwired: 1 in, 1 out]
                        n2642 = local write "Flag Stop"(TRUE ("Flag Stop")) -> ()
                        n2643 = local write "M_AH"(w3250) -> ()
                        n2644 = local write "M_DEC"(w3250) -> ()
                        n2645 = local write "M_CUP"(w3250) -> ()
                        n2646 = local write "M_PROT"(w3250) -> ()
                      }
                      frame #1 {
                        w3252 = FALSE
                        w3253 = u8 0 ("Disabled")
                        # "DESLIGA TODOS"
                        # "HABILITA TODOS"
                        n2647 = local write "BtUtilZenith"(w3252) -> ()
                        n2648 = local write "BtUtilPark"(w3252) -> ()
                        n2649 = local write "FLAT-FIELD"(w3252) -> ()
                        n2650 = local write "PROTEÇÃO"(w3252) -> ()
                        n2651 = local write "ECASS"(w3252) -> ()
                        n2652 = property on="BtUtilPark" class="Bool (strict)"("Disabled"=w3253) -> ()  [unwired: 2 in, 2 out]
                        n2653 = property on="ECASS" class="Bool (strict)"("Disabled"=w3253) -> ()  [unwired: 2 in, 2 out]
                        n2654 = property on="BtUtilZenith" class="Bool (strict)"("Disabled"=w3253) -> ()  [unwired: 2 in, 2 out]
                        n2655 = property on="PROTEÇÃO" class="Bool (strict)"("Disabled"=w3253) -> ()  [unwired: 2 in, 2 out]
                        n2656 = property on="FLAT-FIELD" class="Bool (strict)"("Disabled"=w3253) -> ()  [unwired: 2 in, 2 out]
                      }
                    }
                  }
                }
                n2657 = Compound Arithmetic op=OR("BtUtilPark", "BtUtilZenith", "ECASS", "FLAT-FIELD", "PROTEÇÃO") -> (→"MOVING":bool)
              }
              frame #1 {
                # "MÁQUINAS DE ESTADOS DAS TAMPAS"
                n2658 = case shown="True" "Case Constant\n(See Context Help) 11" {
                  frame False {
                    # "ABRIR"
                    # "FECHAR"
                    n2659 = case shown="\"PIZZA\"" "ESTADO FECHAR" {
                      tunnel: [w3304 w3312 w3323 w3331 w3341 w3349 w3359 "REPOUSO" ("y")] -> w3258
                      frame "INICIO", Default {
                        w3309 = u16 3 items=["ZERO", "AH", "DEC", "TUBO", "CUP"] ("Controlador")
                        # "SELECIONA DISPOSITVO BACIA E\nMANDA FECHAR"
                        # "DISP=1 E PIZZA=1"
                        n2660 = call "Monta Comando.vi"("Set Point"=" A0 A0", "Comando"="ESCREVER", "Dispositivo"="TAMPAS" ("Comando"), "Controlador"=w3309) -> ("Resposta"=w3305:string)  [unwired: 3 in, 2 out]
                        n2661 = Not Equal?(x=w3305, y="TAMPAS OK") -> ()  [unwired: 1 out]
                        n2662 = Tick Count (ms)() -> (millisecond timer value=→"T1 2":u32)
                        n2663 = Select(t="REPOUSO" ("y"), s=FALSE, f="ESPERA 1" ("y")) -> (s? t:f=w3304:string)
                      }
                      frame "ESPERA 1" {
                        # "20 SEGUNDOS"
                        n2664 = local read "T1 2"() -> (w3317:u32)
                        n2665 = Tick Count (ms)() -> (millisecond timer value=w3315:u32)
                        n2666 = Add(x=w3317, y=u32 20000) -> (x+y=w3314:u32)
                        n2667 = Greater?(x=w3315, y=w3314) -> (0:w3311:bool)
                        n2668 = Select(t="PIZZA" ("y"), s=w3311, f="ESPERA 1" ("y")) -> (s? t:f=w3312:string)
                      }
                      frame "PIZZA" {
                        w3328 = u16 3 items=["ZERO", "AH", "DEC", "TUBO", "CUP"] ("Controlador")
                        # "SELECIONA DISP PIZZA\nE MANDA FECHAR"
                        # "PIZZA=1"
                        n2669 = call "Monta Comando.vi"("Set Point"=" 30 10", "Comando"="ESCREVER", "Dispositivo"="TAMPAS" ("Comando"), "Controlador"=w3328) -> ("Resposta"=w3322:string)  [unwired: 3 in, 2 out]
                        n2670 = Tick Count (ms)() -> (millisecond timer value=→"T2 2":u32)
                        n2671 = Not Equal?(x=w3322, y="TAMPAS OK") -> ()  [unwired: 1 out]
                        n2672 = Select(t="REPOUSO" ("y"), s=FALSE, f="PIZZA 2") -> (s? t:f=w3323:string)
                      }
                      frame "PIZZA 2" {
                        w3339 = u16 3 items=["ZERO", "AH", "DEC", "TUBO", "CUP"] ("Controlador")
                        n2673 = call "Monta Comando.vi"("Set Point"=" F8 90", "Comando"="ESCREVER", "Dispositivo"="TAMPAS" ("Comando"), "Controlador"=w3339) -> ("Resposta"=w3334:string)  [unwired: 3 in, 2 out]
                        n2674 = Tick Count (ms)() -> (millisecond timer value=→"T2 3":u32)
                        n2675 = Not Equal?(x=w3334, y="TAMPAS OK") -> ()  [unwired: 1 out]
                        n2676 = Select(t="REPOUSO" ("y"), s=FALSE, f="ESPERA 1A") -> (s? t:f=w3331:string)
                      }
                      frame "ESPERA 1A" {
                        # "2 SEGUNDOS"
                        n2677 = local read "T2 3"() -> (w3344:u32)
                        n2678 = Tick Count (ms)() -> (millisecond timer value=w3346:u32)
                        n2679 = Add(x=w3344, y=u32 2000) -> (x+y=w3347:u32)
                        n2680 = Greater?(x=w3346, y=w3347) -> (0:w3340:bool)
                        n2681 = Select(t="PIZZA 3" ("y"), s=w3340, f="ESPERA 1A" ("y")) -> (s? t:f=w3341:string)
                      }
                      frame "PIZZA 3" {
                        w3357 = u16 3 items=["ZERO", "AH", "DEC", "TUBO", "CUP"] ("Controlador")
                        # "PIZZA=3"
                        n2682 = call "Monta Comando.vi"("Set Point"=" 48 48", "Comando"="ESCREVER", "Dispositivo"="TAMPAS" ("Comando"), "Controlador"=w3357) -> ("Resposta"=w3352:string)  [unwired: 3 in, 2 out]
                        n2683 = Not Equal?(x=w3352, y="TAMPAS OK") -> ()  [unwired: 1 out]
                        n2684 = Select(t="REPOUSO" ("y"), s=FALSE, f="ESPERA 2" ("y")) -> (s? t:f=w3349:string)
                      }
                      frame "ESPERA 2" {
                        # "10 SEGUNDOS"
                        n2685 = local read "T2 2"() -> (w3363:u32)
                        n2686 = Tick Count (ms)() -> (millisecond timer value=w3361:u32)
                        n2687 = Add(x=w3363, y=u32 10000) -> (x+y=w3360:u32)
                        n2688 = Greater?(x=w3361, y=w3360) -> (0:w3358:bool)
                        n2689 = case shown="True" w3358 {
                          frame False {
                          }
                          frame True {
                            n2690 = local write "LED ACTION"(FALSE ("LED ACTION")) -> ()
                          }
                        }
                        n2691 = Select(t="REPOUSO" ("y"), s=w3358, f="ESPERA 2" ("y")) -> (s? t:f=w3359:string)
                      }
                      frame "REPOUSO" {
                      }
                    }
                    n2692 = local write "ESTADO FECHAR"(w3258) -> ()
                    n2693 = case shown="\"INICIO\", Default" "ESTADO ABRIR" {
                      tunnel: [w3263 w3272 w3283 w3290 "REPOUSO" ("y")] -> w3256
                      frame "INICIO", Default {
                        w3269 = u16 3 items=["ZERO", "AH", "DEC", "TUBO", "CUP"] ("Controlador")
                        # "SELECIONA DISPOSITVO PIZZA E\nMANDA ABRIR"
                        # "DISP=0 E PIZZA=0"
                        n2694 = call "Monta Comando.vi"("Set Point"=" 30 00", "Comando"="ESCREVER", "Dispositivo"="TAMPAS" ("Comando"), "Controlador"=w3269) -> ("Resposta"=w3264:string)  [unwired: 3 in, 2 out]
                        n2695 = Not Equal?(x=w3264, y="TAMPAS OK") -> ()  [unwired: 1 out]
                        n2696 = Tick Count (ms)() -> (millisecond timer value=→"T1":u32)
                        n2697 = Select(t="REPOUSO" ("y"), s=FALSE, f="ESPERA 1" ("y")) -> (s? t:f=w3263:string)
                      }
                      frame "ESPERA 1" {
                        # "10 SEGUNDOS"
                        n2698 = local read "T1"() -> (w3277:u32)
                        n2699 = Tick Count (ms)() -> (millisecond timer value=w3275:u32)
                        n2700 = Add(x=w3277, y=u32 10000) -> (x+y=w3274:u32)
                        n2701 = Greater?(x=w3275, y=w3274) -> (0:w3271:bool)
                        n2702 = Select(t="BACIA" ("y"), s=w3271, f="ESPERA 1" ("y")) -> (s? t:f=w3272:string)
                      }
                      frame "BACIA" {
                        w3288 = u16 3 items=["ZERO", "AH", "DEC", "TUBO", "CUP"] ("Controlador")
                        # "SELECIONA DISP BACIA\nE MANDA ABRIR"
                        # "BACIA=0"
                        n2703 = call "Monta Comando.vi"("Set Point"=" A0 20", "Comando"="ESCREVER", "Dispositivo"="TAMPAS" ("Comando"), "Controlador"=w3288) -> ("Resposta"=w3282:string)  [unwired: 3 in, 2 out]
                        n2704 = Tick Count (ms)() -> (millisecond timer value=→"T2":u32)
                        n2705 = Not Equal?(x=w3282, y="TAMPAS OK") -> ()  [unwired: 1 out]
                        n2706 = Select(t="REPOUSO" ("y"), s=FALSE, f="ESPERA 2") -> (s? t:f=w3283:string)
                      }
                      frame "ESPERA 2" {
                        # "25 SEGUNDOS"
                        n2707 = local read "T2"() -> (w3294:u32)
                        n2708 = Tick Count (ms)() -> (millisecond timer value=w3292:u32)
                        n2709 = Add(x=w3294, y=u32 25000) -> (x+y=w3291:u32)
                        n2710 = Greater?(x=w3292, y=w3291) -> (0:w3289:bool)
                        n2711 = case shown="True" w3289 {
                          frame False {
                          }
                          frame True {
                            n2712 = local write "LED ACTION"(TRUE ("LED ACTION")) -> ()
                          }
                        }
                        n2713 = Select(t="REPOUSO" ("y"), s=w3289, f="ESPERA 2" ("y")) -> (s? t:f=w3290:string)
                      }
                      frame "REPOUSO" {
                      }
                    }
                    n2714 = local write "ESTADO ABRIR"(w3256) -> ()
                  }
                  frame True {
                    # "NOVO"
                    # "ABRIR"
                    # "FECHAR"
                    n2715 = local read "ESTADO FECHAR"() -> (w3371:string)
                    n2716 = case shown="\"PIZZA3\"" w3371 {
                      tunnel: [w3436 w3444 w3455 w3463 w3471 "REPOUSO" ("y")] -> w3370
                      frame "INICIO", Default {
                        w3441 = u16 3 items=["ZERO", "AH", "DEC", "TUBO", "CUP"] ("Controlador")
                        # "SELECIONA DISPOSITVO BACIA E\nMANDA FECHAR"
                        n2717 = call "Monta Comando.vi"("Set Point"=" A0 A0", "Comando"="ESCREVER", "Dispositivo"="TAMPAS" ("Comando"), "Controlador"=w3441) -> ("Resposta"=w3437:string)  [unwired: 3 in, 2 out]
                        n2718 = Not Equal?(x=w3437, y="TAMPAS OK") -> ()  [unwired: 1 out]
                        n2719 = Tick Count (ms)() -> (millisecond timer value=→"TF1":u32)
                        n2720 = Select(t="REPOUSO" ("y"), s=FALSE, f="ESPERA1" ("y")) -> (s? t:f=w3436:string)
                      }
                      frame "ESPERA1" {
                        # "20 SEGUNDOS"
                        n2721 = local read "TF1"() -> (w3449:u32)
                        n2722 = Tick Count (ms)() -> (millisecond timer value=w3447:u32)
                        n2723 = Add(x=w3449, y=u32 20000) -> (x+y=w3446:u32)
                        n2724 = Greater?(x=w3447, y=w3446) -> (0:w3443:bool)
                        n2725 = Select(t="PIZZA" ("y"), s=w3443, f="ESPERA1" ("y")) -> (s? t:f=w3444:string)
                      }
                      frame "PIZZA" {
                        w3460 = u16 3 items=["ZERO", "AH", "DEC", "TUBO", "CUP"] ("Controlador")
                        # "PASSA PARA MODO\nHANDSET E PIZZA FECHA"
